vi "Fault_Abnormal_state.vi"() -> ()   [LabVIEW 2016]
doc: "-----------------------------------------------------------------------------------------------------------------------\nCopyright <2019> <The University of Tennessee at Knoxville and the University of Tennessee Research Foundation>\nThis software is released under BSD-3 \nhttps://opensource.org/licenses/BSD-3-Clause \nAdditional license options available at https://utrf.tennessee.edu/industry/sample-agreements/\n-----------------------------------------------------------------------------------------------------------------------"
panel:
  out "Function enable by fault/abnormal":bool[](array[boolean])
  out "Error State":errorcluster[](array[cluster])
  in  "Abnormal state flag":bool
  in  "Fault state flag":bool
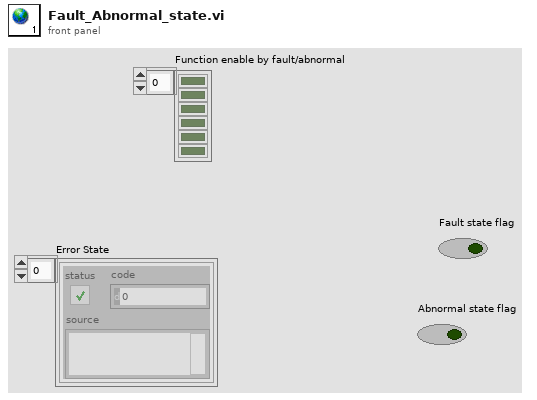
[diagram p1: front panel]
diagram:
